vi "VWflipperArray.vi"(4 "Probe Orientation":u16(ring)=90 items=["Horizontal"=0, "Diagonal"=45, "Vertical"=90, "User Defined"=999], 6 "Probe Type":u16(ring)=5 items=["5-Hole Probe"=5, "OmniProbe"=12], 7 "Theta Degree":dbl[](array[numeric]), 8 "Probe w m/s":dbl[](array[numeric]), 9 "Probe v m/s":dbl[](array[numeric]), 10 "Probe u  m/s":dbl[](array[numeric]), 11 "VMagn m/s":dbl[](array[numeric])) -> (3 "VmagUVWCone":dbl[][](array[numeric]))   [LabVIEW 2016]
uses:
  <vilib>/Analysis/coordinate.llb/Euler Rotation Order.ctl
  <vilib>/Analysis/coordinate.llb/3D Cartesian Coordinate Rotation (Euler) (Array).vi
  <vilib>/Analysis/NI_AALPro.lvlib
panel:
  in  "User-Defined Euler Angles":cluster{"phi":dbl, "theta":dbl, "psi":dbl}
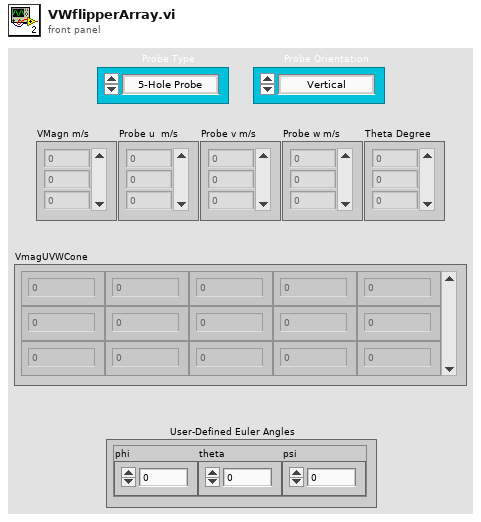
[diagram p1: front panel]
types:
  T1 = typedef "NI_AALPro.lvlib/Euler Rotation Order.ctl" = u16
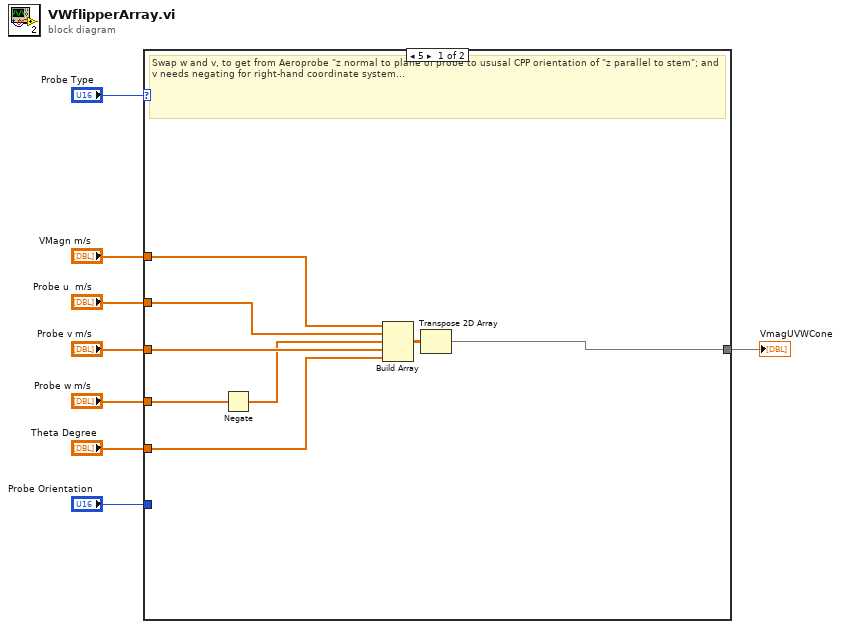
[diagram p0: block diagram]
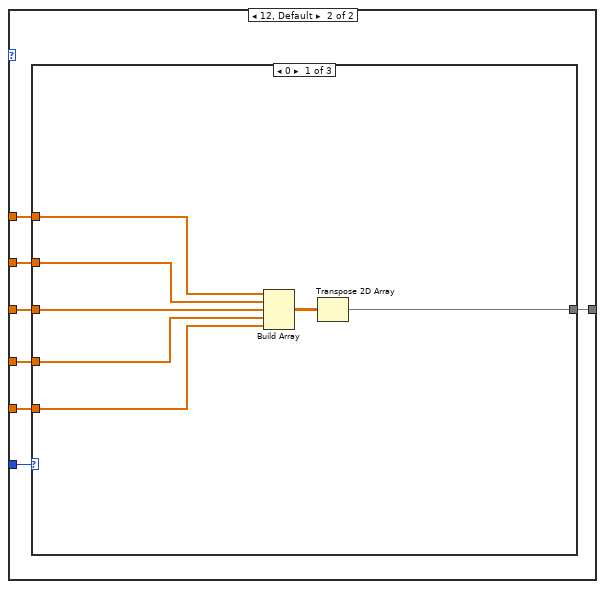
[diagram p2: hidden frame]
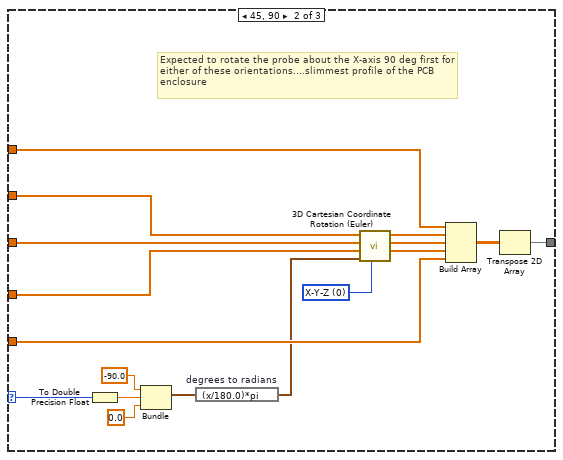
[diagram p3: hidden frame]
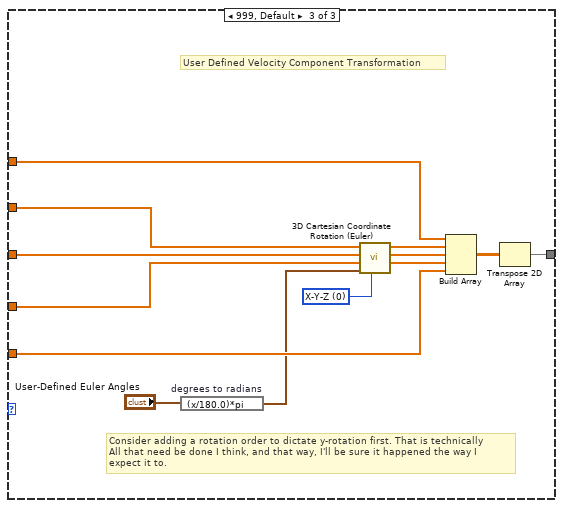
[diagram p4: hidden frame]
diagram:
  n1 = case shown="5" "Probe Type" {
    tunnel: "Theta Degree" -> [w16 w23]
    tunnel: "Probe w m/s" -> [w15 w18]
    tunnel: "Probe v m/s" -> [w14 w19]
    tunnel: "Probe u  m/s" -> [w12 w22]
    tunnel: "VMagn m/s" -> [w11 w21]
    tunnel: [w9 w20] -> w3
    tunnel: "Probe Orientation" -> [_ w17]
    frame 5 {
      # "Swap w and v, to get from Aeroprobe \"z normal to plane of probe to ususal CPP orientation of \"z parallel to stem\"; and v needs negating for right-hand coordinate system..."
      n2 = Negate(x=w15) -> (-x=w13:dbl[])
      n3 = Build Array(w11, w12, w13, w14, w16) -> (w10:dbl[][])
      n4 = Transpose 2D Array(2D array=w10) -> (transposed array=w9:dbl[][])
    }
    frame 12, Default {
      n5 = case shown="0" w17 {
        selector: w17 -> [_ w40 _]
        tunnel: w23 -> [w30 w47 w60]
        tunnel: w22 -> [w29 w42 w55]
        tunnel: w21 -> [w28 w46 w59]
        tunnel: [w26 w44 w57] -> w20
        tunnel: w19 -> [w25 w43 w56]
        tunnel: w18 -> [w24 w41 w54]
        frame 0 {
          n6 = Build Array(w28, w29, w25, w24, w30) -> (w27:dbl[][])
          n7 = Transpose 2D Array(2D array=w27) -> (transposed array=w26:dbl[][])
        }
        frame 45, 90 {
          w36 = T1 0 items=["X-Y-Z", "X-Z-Y", "Y-X-Z", "Y-Z-X", "Z-X-Y", "Z-Y-X", "X-Y-X", "X-Z-X", "Y-X-Y", "Y-Z-Y", "Z-X-Z", "Z-Y-Z"] ("rotation order")
          # "Expected to rotate the probe about the X-axis 90 deg first for either of these orientations....slimmest profile of the PCB enclosure"
          n8 = To Double Precision Float(number=w40) -> (double precision float=w33:dbl)
          n9 = Bundle("phi"=-90.0, w33, "theta"=0.0) -> (w32:cluster{"phi":dbl, dbl, "theta":dbl})  [unwired: 1 in]
          n10 = expression code="(x/180.0)*pi" "degrees to radians"(w32) -> (w31:cluster{"phi":dbl, dbl, "theta":dbl})
          n11 = call-poly <vilib>:"3D Cartesian Coordinate Rotation (Euler).vi"("rotation order"=w36, "Euler Angles"=w31, "Z"=w41, "Y"=w43, "X"=w42) -> ("Z Out"=w37:dbl[], "Y Out"=w38:dbl[], "X Out"=w39:dbl[])  [unwired: 3 in, 1 out]
          n12 = Build Array(w46, w39, w38, w37, w47) -> (w45:dbl[][])
          n13 = Transpose 2D Array(2D array=w45) -> (transposed array=w44:dbl[][])
        }
        frame 999, Default {
          w50 = T1 0 items=["X-Y-Z", "X-Z-Y", "Y-X-Z", "Y-Z-X", "Z-X-Y", "Z-Y-X", "X-Y-X", "X-Z-X", "Y-X-Y", "Y-Z-Y", "Z-X-Z", "Z-Y-Z"] ("rotation order")
          # "User Defined Velocity Component Transformation"
          # "Consider adding a rotation order to dictate y-rotation first. That is technically\nAll that need be done I think, and that way, I'll be sure it happened the way I\nexpect it to."
          n14 = expression code="(x/180.0)*pi" "degrees to radians"("User-Defined Euler Angles") -> (w48:cluster{"phi":dbl, "theta":dbl, "psi":dbl})
          n15 = call-poly <vilib>:"3D Cartesian Coordinate Rotation (Euler).vi"("rotation order"=w50, "Euler Angles"=w48, "Z"=w54, "Y"=w56, "X"=w55) -> ("Z Out"=w51:dbl[], "Y Out"=w52:dbl[], "X Out"=w53:dbl[])  [unwired: 3 in, 1 out]
          n16 = Build Array(w59, w53, w52, w51, w60) -> (w58:dbl[][])
          n17 = Transpose 2D Array(2D array=w58) -> (transposed array=w57:dbl[][])
        }
      }
    }
  }
  "VmagUVWCone" <- w3
